vi "MAIN_ALL_TEST.vi"() -> ()   [LabVIEW 2016]
uses:
  System.Windows.Forms
  <vilib>/picture/picture.llb/imagedata.ctl
  System.Drawing
  <vilib>/wsapi/NI_WebServices.lvlib
  USER32.DLL
  <vilib>/Utility/importsl/GetValueByPointer/datatype.ctl
  <vilib>/Utility/importsl/GetValueByPointer/GetValueByPointer.xnode
  <resource>/lvimptsl.dll
panel:
  in  "Pointer":u64
  out "Output":i32
  in  "ErrorIn":errorcluster
  out "ErrorOut":errorcluster
  out "Value":i32
  in  "Address (Pointer)":i64
  in  "error in (no error) 2":errorcluster
  out "error out":errorcluster
  out "hWnd":u32
  out "hWnd 2":u32
  out "error out 2":errorcluster
  out "hWnd 3":u32
  out "speed":dbl
  out "return type":i32
  out "IMAQ Image":T1(plugin-control)
  in  "PictureBox":refnum<k24>(container)
  out "VLC media player pointer (p_mi)":i32
  out "VLC media pointer (p_md)":i32
  out "VLC Istance pointer (p_instance)":i32
  in  "error in (no error)":errorcluster
  in  "Media Source":string="rtsp://admin:admin8@192.168.1.108/cam/realmonitor?channel=1&subtype=0"
  in  "Script":string
  # "rtsp://admin:gamma2018@84.253.163.35/cam/realmonitor?channel=1&subtype=1"
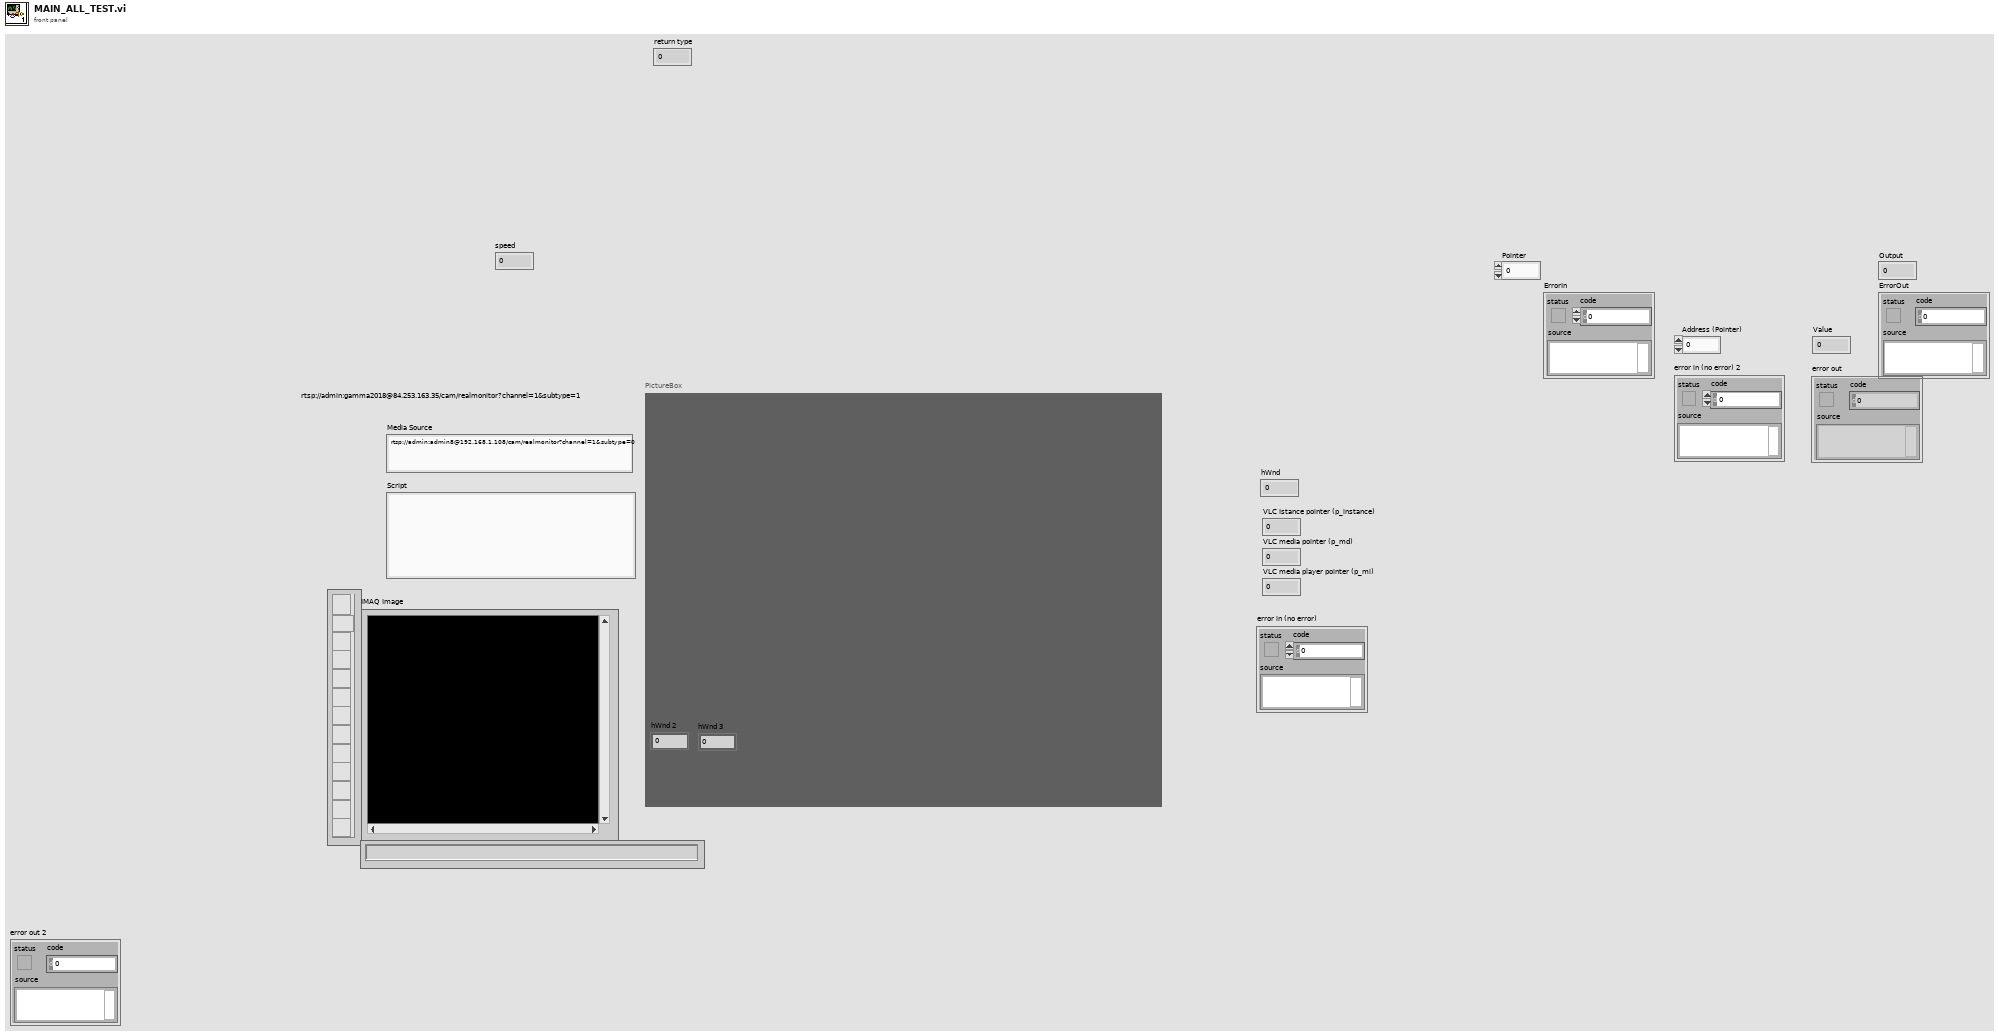
[diagram p1: front panel]
types:
  T1 = typedef "IMAQ Image.ctl" = refnum<image>
  T2 = typedef "Image Type" = u32
  T3 = typedef "imagedata.ctl" = cluster{"image type":i32, "image depth":i32, "image":u8[], "mask":u8[], "colors":u32[], "Rectangle":cluster{"left":i16, "top":i16, "right":i16, "bottom":i16}}
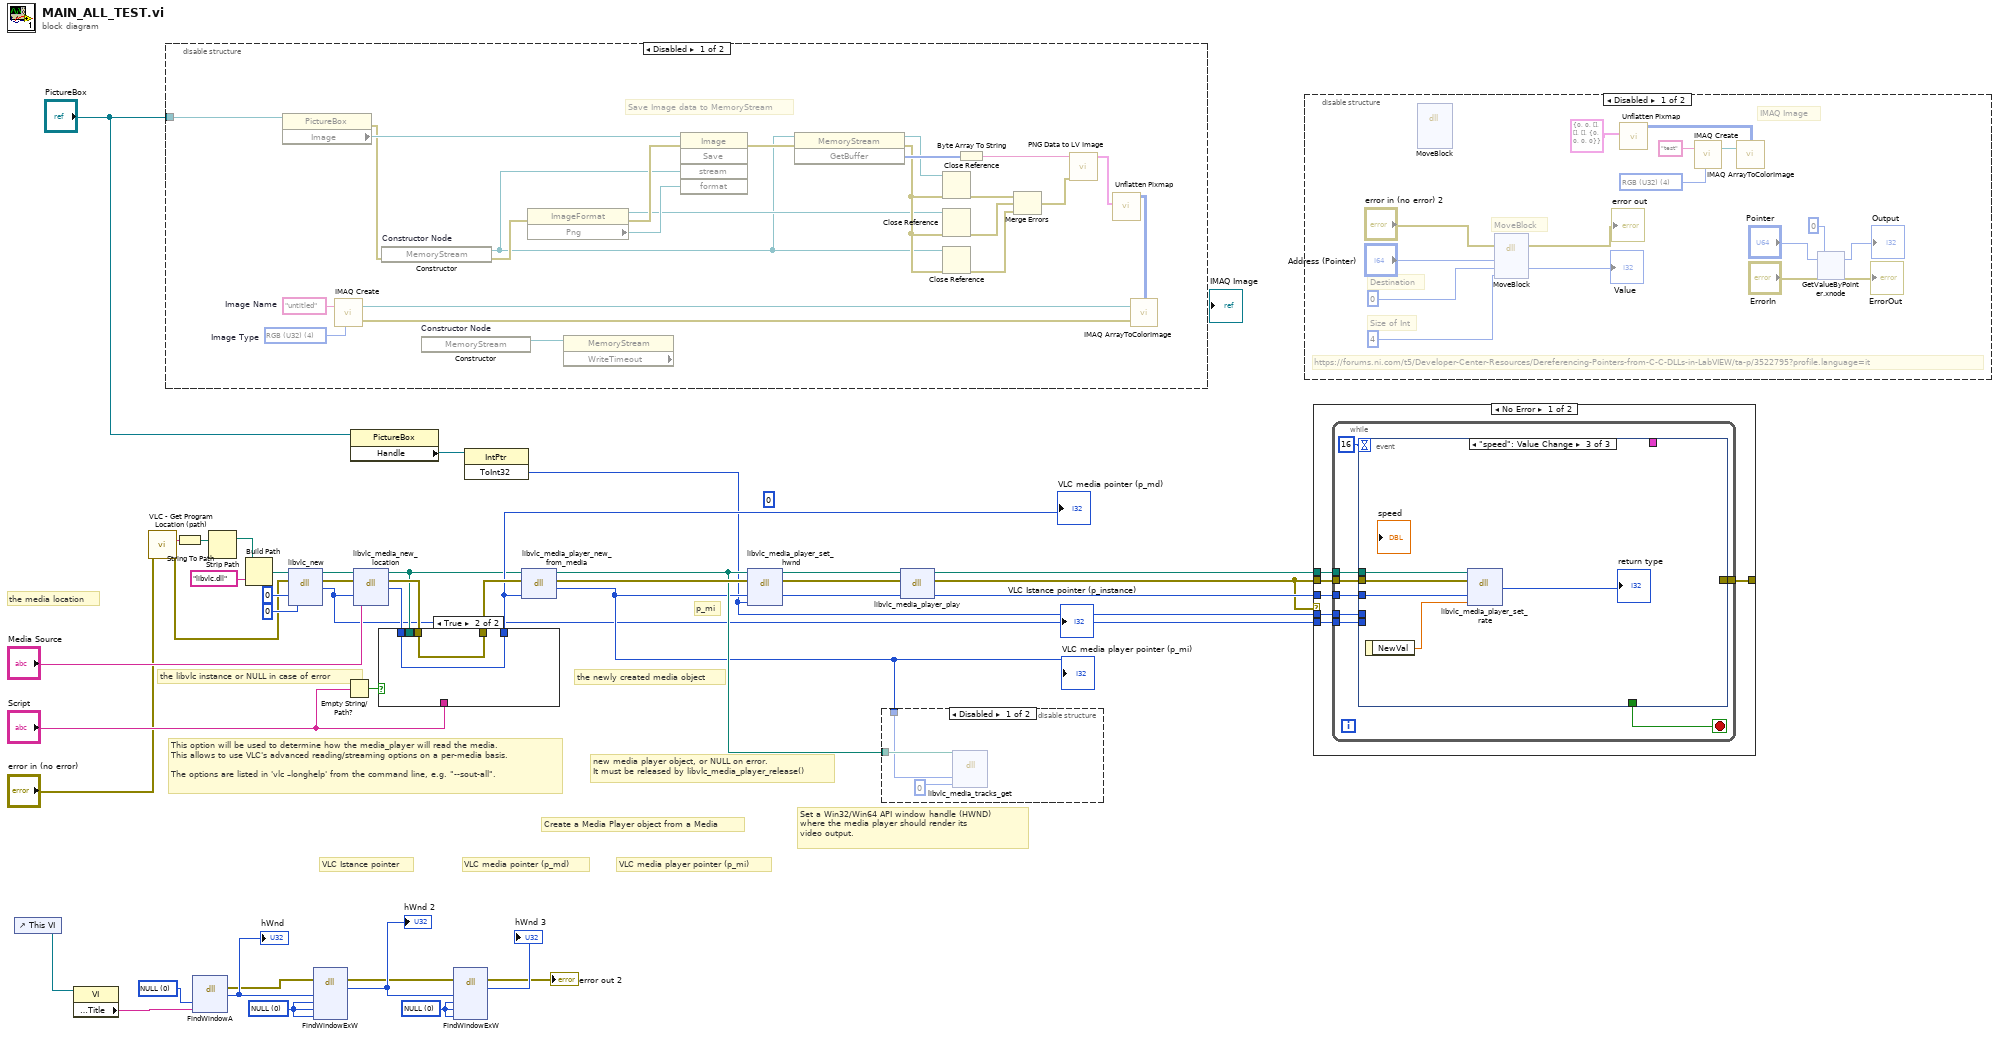
[diagram p0: block diagram]
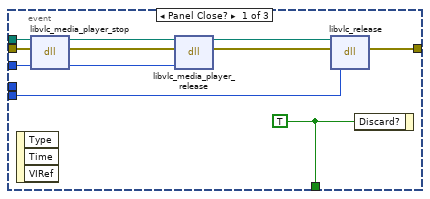
[diagram p3: hidden frame]
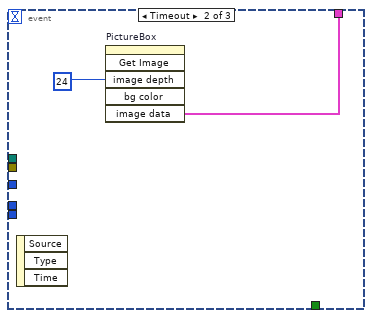
[diagram p4: hidden frame]
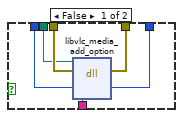
[diagram p8: hidden frame]
diagram:
  w7 = 0 items=["NULL"]
  w3 = 0 items=["NULL"]
  w1 = 0 items=["NULL"]
  (unwired) 0 ("ToInt32")
  # "VLC media player pointer (p_mi)"
  # "VLC media pointer (p_md)"
  # "VLC Istance pointer"
  # "p_mi"
  # "Set a Win32/Win64 API window handle (HWND) \nwhere the media player should render its \nvideo output."
  # "new media player object, or NULL on error. \nIt must be released by libvlc_media_player_release()"
  # "Create a Media Player object from a Media"
  # "This option will be used to determine how the media_player will read the media. \nThis allows to use VLC's advanced reading/streaming options on a per-media basis.\n\nThe options are listed in 'vlc –longhelp' from the command line, e.g. \"--sout-all\"."
  # "the newly created media object"
  # "the media location"
  # "the libvlc instance or NULL in case of error"
  n1 = control-ref of="This VI"() -> (w11:refnum<vi>)
  n2 = property class="VI"(reference=w11) -> ("Front Panel Window:Title"=w2:string)  [unwired: 1 in, 2 out]
  n3 = call "VLC - Get Program Location (path).vi"("error in (no error)"="error in (no error)") -> ("VLC path"=w33:string, "error out"=w28:errorcluster)  [unwired: 13 in]
  n4 = disable-structure shown="Disabled" {
    disable-tunnel: "PictureBox" -> [w44 _]
    frame Disabled {
      w67 = "untitled"  # Image Name
      w66 = T2 4 items=["Grayscale (U8)", "Grayscale (I16)", "Grayscale (SGL)", "Complex (CSG)", "RGB (U32)", "HSL (U32)", "RGB (U64)", "Grayscale (U16)"]  # Image Type
      # "Save Image data to MemoryStream"
      n5 = property class="PictureBox"(reference=w44) -> (error out=w55:errorcluster, "Image"=w63:refnum<k24>)  [unwired: 1 in, 1 out]
      n6 = call "IMAQ Create"("Image Name"=w67, "Image Type"=w66) -> ("New Image"=w65:T1, "error out"=w46:errorcluster)  [unwired: 3 in]
      n7 = constructor on="Constructor Node" class="MemoryStream"(error in=w55) -> (reference out=w51:refnum<k24>, error out=w57:errorcluster)  [unwired: 2 in, 1 out]
      n8 = constructor on="Constructor Node" class="MemoryStream"() -> (reference out=w45:refnum<k24>)  [unwired: 3 in, 2 out]
      n9 = property class="ImageFormat"(error in=w57) -> (reference out=w52:refnum<k24>, error out=w56:errorcluster, "Png"=w59:refnum<k24>)  [unwired: 1 in]
      n10 = property class="MemoryStream" props=["WriteTimeout"](reference=w45) -> ()  [unwired: 1 in, 3 out]
      n11 = invoke class="Image" method="Save"(reference=w63, error in=w56, "stream"=w51, "format"=w59) -> (error out=w58:errorcluster)  [unwired: 1 in, 4 out]
      n12 = invoke class="MemoryStream" method="GetBuffer"(reference=w51, error in=w58) -> (reference out=w54:refnum<k24>, error out=w53:errorcluster, "GetBuffer"=w61:u8[])  [unwired: 1 in]
      n13 = Close Reference(reference=w54, error in (no error)=w53) -> (error out=w50:errorcluster)
      n14 = Close Reference(reference=w52, error in (no error)=w53) -> (error out=w49:errorcluster)
      n15 = Close Reference(reference=w51, error in (no error)=w53) -> (error out=w48:errorcluster)
      n16 = Byte Array To String(unsigned byte array=w61) -> (string=w60:string)
      n17 = Merge Errors "Merge Errors"(w50, w49, w48) -> (w47:errorcluster)
      n18 = call <vilib>:"PNG Data to LV Image.vi"("error in (no error)"=w47, "png data"=w60) -> ("image data"=w62:T3)  [unwired: 8 in, 1 out]
      n19 = call <vilib>:"Unflatten Pixmap.vi"("image data"=w62) -> ("24-bit pixmap"=w64:u32[][])  [unwired: 4 in, 6 out]
      n20 = call "IMAQ ArrayToColorImage"("Image Pixels (U32)"=w64, "Image"=w65, "error in (no error)"=w46) -> ()  [unwired: 2 in, 2 out]
    }
    frame Enabled {
    }
  }
  n21 = String To Path(string=w33) -> (path=w32:path)
  n22 = dll-call lib="USER32.DLL" fn="FindWindowA" label="FindWindow"("lpszClassName"=w1, "lpszWindowName"=w2) -> (error out=w4:errorcluster, "hWnd"=w10:u32)  [unwired: 5 in, 1 out]
  "hWnd" <- w10
  n23 = Strip Path(path=w32) -> (stripped path=w22:path)  [unwired: 1 out]
  n24 = Build Path(base path=w22, name or relative path="libvlc.dll") -> (appended path=w30:path)
  n25 = dll-call lib="C:/Program Files (x86)/VideoLAN/VLC/libvlc.dll" fn="libvlc_new"(path in=w30, error in=w28, "argc"=i16 0, "argv"=u8 0) -> (path out=w35:path, error out=w38:errorcluster, "return type"=w15:i32)  [unwired: 3 in]
  "VLC Istance pointer (p_instance)" <- w15
  n26 = dll-call lib="user32.dll" fn="FindWindowExW" label="FindWindowEx"(error in=w4, "hwndParent"=w10, "hwndChildAfter"=w3, "lpszClassName"=w3, "lpszWindowName"=w3) -> (error out=w5:errorcluster, "hWnd"=w6:u32)  [unwired: 6 in, 1 out]
  "hWnd 2" <- w6
  n27 = Empty String/Path?(string/path="Script") -> (empty?=w26:bool)
  n28 = property class="PictureBox"(reference="PictureBox") -> ("Handle"=w14:refnum<k24>)  [unwired: 1 in, 2 out]
  n29 = dll-call lib="C:/Program Files (x86)/VideoLAN/VLC/libvlc.dll" fn="libvlc_media_new_location"(path in=w35, error in=w38, "p_instance"=w15, "path"="Media Source") -> (path out=w25:path, error out=w40:errorcluster, "return type"=w41:i32)  [unwired: 3 in]
  n30 = case shown="True" w26 {
    tunnel: w40 -> [w73 w75]
    tunnel: w41 -> [w72 w74]
    tunnel: [w71 w74] -> w42
    tunnel: [w70 w75] -> w43
    tunnel: "Script" -> [w69 _]
    tunnel: w25 -> [w68 _]
    frame False {
      n31 = dll-call lib="C:/Program Files (x86)/VideoLAN/VLC/libvlc.dll" fn="libvlc_media_add_option"(path in=w68, error in=w73, "p_md"=w72, "ppsz_options"=w69) -> (error out=w70:errorcluster, "p_md"=w71:i32)  [unwired: 3 in, 1 out]
    }
    frame True {
    }
  }
  "VLC media pointer (p_md)" <- w42
  n32 = dll-call lib="user32.dll" fn="FindWindowExW" label="FindWindowEx"(error in=w5, "hwndParent"=w6, "hwndChildAfter"=w7, "lpszClassName"=w7, "lpszWindowName"=w7) -> (error out=→"error out 2":errorcluster, "hWnd"=→"hWnd 3":u32)  [unwired: 6 in, 1 out]
  n33 = invoke class="IntPtr" method="ToInt32"(reference=w14) -> ("ToInt32"=w12:i32)  [unwired: 2 in, 2 out]
  n34 = dll-call lib="C:/Program Files (x86)/VideoLAN/VLC/libvlc.dll" fn="libvlc_media_player_new_from_media"(path in=w25, error in=w43, "p_md"=w42) -> (path out=w20:path, error out=w39:errorcluster, "return type"=w19:i32)  [unwired: 2 in]
  "VLC media player pointer (p_mi)" <- w19
  n35 = dll-call lib="C:/Program Files (x86)/VideoLAN/VLC/libvlc.dll" fn="libvlc_media_player_set_hwnd"(path in=w20, error in=w39, "p_mi"=w19, "drawable"=w12) -> (path out=w34:path, error out=w23:errorcluster, "p_mi"=w24:i32)  [unwired: 3 in]
  n36 = disable-structure shown="Disabled" {
    disable-tunnel: w20 -> [w78 _]
    disable-tunnel: w19 -> [w77 _]
    frame Disabled {
      n37 = dll-call lib="C:/Program Files (x86)/VideoLAN/VLC/libvlc.dll" fn="libvlc_media_tracks_get"(path in=w78, "p_mi"=w77, "drawable"=0 ("ToInt32")) -> ()  [unwired: 5 in, 2 out]
    }
    frame Enabled {
    }
  }
  n38 = dll-call lib="C:/Program Files (x86)/VideoLAN/VLC/libvlc.dll" fn="libvlc_media_player_play"(path in=w34, error in=w23, "p_mi"=w24) -> (path out=w18:path, error out=w16:errorcluster, "p_mi"=w17:i32)  [unwired: 2 in]
  n39 = disable-structure shown="Disabled" {
    frame Disabled {
      w92 = T2 4 items=["Grayscale (U8)", "Grayscale (I16)", "Grayscale (SGL)", "Complex (CSG)", "RGB (U32)", "HSL (U32)", "RGB (U64)", "Grayscale (U16)"] ("Image Type")
      # "https://forums.ni.com/t5/Developer-Center-Resources/Dereferencing-Pointers-from-C-C-DLLs-in-LabVIEW/ta-p/3522795?profile.language=it"
      # "Destination"
      # "Size of Int"
      # "MoveBlock"
      # "IMAQ Image"
      n40 = dll-call lib="LabVIEW" fn="MoveBlock"() -> ()  [unwired: 10 in, 2 out]
      n41 = dll-call lib="LabVIEW" fn="MoveBlock"(error in="error in (no error) 2", "Address (Pointer)"="Address (Pointer)", "Destination"=0, "Size"=4 ("arg3")) -> (error out=→"error out":errorcluster, "Destination"=→"Value":i32)  [unwired: 5 in, 1 out]
      n42 = call <vilib>:"Unflatten Pixmap.vi"("image data"=T3 {"image type"=0, "image depth"=0, "image"=[], "mask"=[], "colors"=[], "Rectangle"={"left"=0, "top"=0, "right"=0, "bottom"=0}}) -> ("24-bit pixmap"=w93:u32[][])  [unwired: 4 in, 6 out]
      n43 = call "IMAQ Create"("Image Name"="test", "Image Type"=w92) -> ("New Image"=w90:T1)  [unwired: 3 in, 1 out]
      n44 = call "IMAQ ArrayToColorImage"("Image Pixels (U32)"=w93, "Image"=w90) -> ()  [unwired: 3 in, 2 out]
      n45 = xnode "GetValueByPointer.xnode"("Pointer"="Pointer", "InputType"=0, "ErrorIn"="ErrorIn") -> ("Output"=→"Output":i32, "ErrorOut"=→"ErrorOut":errorcluster)  [unwired: 1 in]
    }
    frame Enabled {
    }
  }
  n46 = case shown="No Error" w16 {
    tunnel: w15 -> [w108 _]
    tunnel: w17 -> [w107 _]
    tunnel: w16 -> [w106 w135]
    tunnel: w18 -> [w105 _]
    tunnel: [w104 w135] -> _
    tunnel: w12 -> [w103 _]
    frame No Error {
      n47 = while {
        tunnel: w108 -> [w116]
        tunnel: w107 -> [w115]
        tunnel: w106 -> [w114]
        tunnel: w105 -> [w113]
        tunnel: [w112] -> w104
        tunnel: w103 -> [w109]
        stop <- w111 stop-if-true
        n48 = event shown="[2] \"speed\": Value Change" {
          selector: _ -> [_ _ _]
          dyn-events: _ -> [_ _ _]
          timeout: 16 -> [_ _ _]
          tunnel: w114 -> [w127 _ w133]
          tunnel: w115 -> [w126 _ w132]
          tunnel: w116 -> [w122 _ _]
          tunnel: w113 -> [w121 _ w134]
          tunnel: [w118 _ _] -> w112
          tunnel: [w117 _ _] -> w111
          tunnel: w109 -> [_ _ _]
          tunnel: [_ w128 _] -> _
          event Panel Close? {
            w117 = TRUE ("Discard?")
            n49 = event-data() -> ()  [unwired: 1 in, 3 out]
            n50 = dll-call lib="C:/Program Files (x86)/VideoLAN/VLC/libvlc.dll" fn="libvlc_media_player_stop"(path in=w121, error in=w127, "p_mi"=w126) -> (path out=w120:path, error out=w125:errorcluster, "p_mi"=w124:i32)  [unwired: 2 in]
            n51 = dll-call lib="C:/Program Files (x86)/VideoLAN/VLC/libvlc.dll" fn="libvlc_media_player_release"(path in=w120, error in=w125, "p_mi"=w124) -> (path out=w119:path, error out=w123:errorcluster)  [unwired: 3 in]
            n52 = dll-call lib="C:/Program Files (x86)/VideoLAN/VLC/libvlc.dll" fn="libvlc_release"(path in=w119, error in=w123, "p_instnace"=w122) -> (error out=w118:errorcluster)  [unwired: 3 in, 1 out]
            n53 = event-data("Discard?"=w117) -> ()  [unwired: 1 in, 1 out]
          }
          event Timeout {
            n54 = event-data() -> ()  [unwired: 1 in, 3 out]
            n55 = invoke on="PictureBox" class="AXCont" method="Get Image"("image depth"=24 ("Image Depth")) -> ("image data"=w128:T3)  [unwired: 5 in, 5 out]
          }
          event "speed": Value Change {
            n56 = event-data() -> ("NewVal"=w131:dbl)  [unwired: 1 in]
            n57 = dll-call lib="C:/Program Files (x86)/VideoLAN/VLC/libvlc.dll" fn="libvlc_media_player_set_rate"(path in=w134, error in=w133, "p_mi"=w132, "rate"=w131) -> ("return type"=→"return type":i32)  [unwired: 3 in, 2 out]
          }
        }
      }
    }
    frame Error {
    }
  }
